vi "Default Configuration--constant.vi"() -> (3 "Default Configuration":T1)   [LabVIEW 2020, in "CML UI.lvlib" / "Configuration.lvclass"]
doc: "This VI stores the default configuration for the module, used when there is no stored config, or the user wants to restore the config to default values.\n____\nPeloton Config 2.0.0.9\nCopyright (c) 2024, Peloton"
uses:
  Configuration.lvclass
  Configuration--cluster.ctl
  Configuration.lvclass/Configuration.ctl
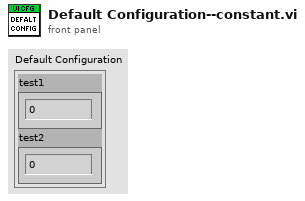
[diagram p1: front panel]
types:
  T1 = typedef "CML UI.lvlib/Configuration.lvclass/Configuration--cluster.ctl" = cluster{"test1":dbl, "test2":dbl}
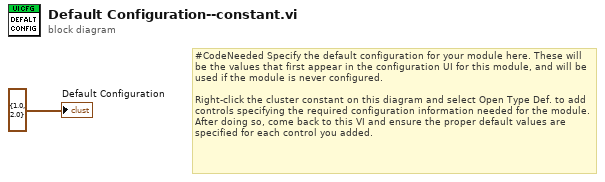
[diagram p0: block diagram]
diagram:
  # "#CodeNeeded Specify the default configuration for your module here. These will be the values that first appear in the configuration UI for this module, and will be used if the module is never configured.\n\nRight-click the cluster constant on this diagram and select Open Type Def. to add controls specifying the required configuration information needed for the module. After doing so, come back to this VI and ensure the proper default values are specified for each control you added."
  "Default Configuration" <- T1 {"test1"=1.0, "test2"=2.0} ("Default Configuration")
